vi "sc5511a_get_rf_parameters.vi"(0 "deviceHandle":u32 format="%.0x", 5 "error in":errorcluster) -> (14 "deviceHandle":u32 format="%.0x", 16 "RF Params":T1 {"RF1 Level (dBm)" format="%.2g"}, 19 "error out":errorcluster)   [LabVIEW 2010]
uses:
  sc5511a.dll
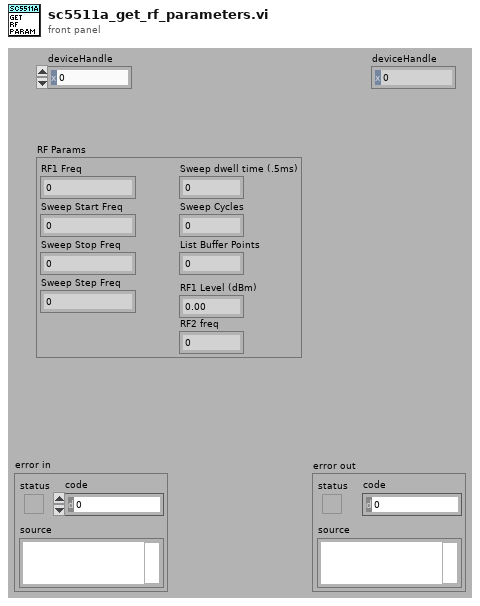
[diagram p1: front panel]
types:
  T1 = cluster{"RF1 Freq":u64, "Sweep Start Freq":u64, "Sweep Stop Freq":u64, "Sweep Step Freq":u64, "Sweep dwell time (.5ms)":u32, "Sweep Cycles":u32, "List Buffer Points":u32, "RF1 Level (dBm)":sgl, "RF2 freq":u16}
  T2 = cluster{"RF1 Freq":u64, "Sweep Start Freq":u64, "Sweep Stop Freq":u64, "Sweep Step Freq":u64, "Sweep dwell time (.5ms)":u32, "Sweep Cycles":u32, "List Buffer Points":u32, "RF1 Level":sgl, "RF2 freq":u16}
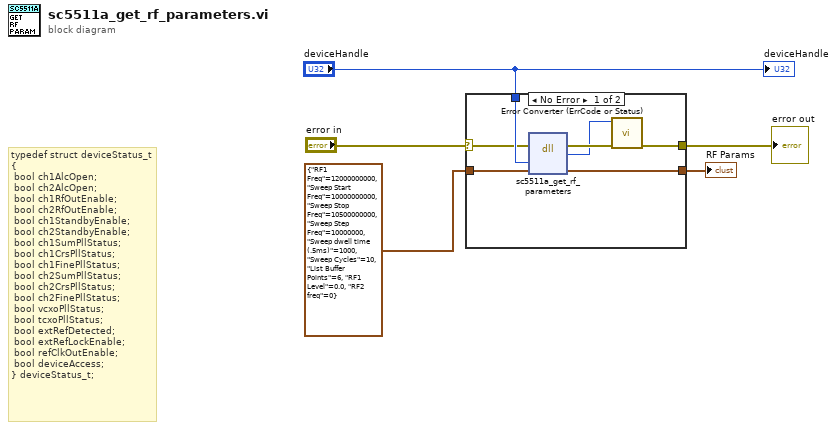
[diagram p0: block diagram]
diagram:
  # "typedef struct deviceStatus_t\n{\n\tbool ch1AlcOpen;\n\tbool ch2AlcOpen;\n\tbool ch1RfOutEnable;\n\tbool ch2RfOutEnable;\n\tbool ch1StandbyEnable;\t\t\t\t\t\n\tbool ch2StandbyEnable;\n\tbool ch1SumPllStatus;\n\tbool ch1CrsPllStatus;\n\tbool ch1FinePllStatus;\n\tbool ch2SumPllStatus;\n\tbool ch2CrsPllStatus;\n\tbool ch2FinePllStatus;\n\tbool vcxoPllStatus;\n\tbool tcxoPllStatus;\n\tbool extRefDetected;\n\tbool extRefLockEnable;\n\tbool refClkOutEnable;\n\tbool deviceAccess;\n}\tdeviceStatus_t;"
  n1 = case shown="No Error" "error in" {
    selector: "error in" -> [w7 w14]
    tunnel: [w12 w14] -> w4
    tunnel: "deviceHandle" -> [w9 _]
    tunnel: T2 {"RF1 Freq"=12000000000, "Sweep Start Freq"=10000000000, "Sweep Stop Freq"=10500000000, "Sweep Step Freq"=10000000, "Sweep dwell time (.5ms)"=1000, "Sweep Cycles"=10, "List Buffer Points"=6, "RF1 Level"=0.0, "RF2 freq"=0} ("RF Params") -> [w8 w13]
    tunnel: [w6 w13] -> w2
    frame No Error {
      n2 = dll-call lib="sc5511a.dll" fn="sc5511a_get_rf_parameters"(error in=w7, "deviceHandle"=w9, "rf_parameters"=w8) -> (error out=w11:errorcluster, "return type"=w10:i32, "rf_parameters"=w6:T2)  [unwired: 3 in, 1 out]
      n3 = call "Error Converter (ErrCode or Status).vi"("error in (no error)"=w11, "error code"=w10) -> ("error out"=w12:errorcluster)  [unwired: 9 in]
    }
    frame Error {
    }
  }
  "error out" <- w4
  "RF Params" <- w2
  "deviceHandle" <- "deviceHandle"
